vi "Is Enum Control.vi"(8 "error in":errorcluster, 11 "control reference in":refnum<vi>) -> (0 "error out":errorcluster, 1 "is enum control":bool, 2 "enum reference out":refnum<vi>, 3 "control reference out":refnum<vi>)   [LabVIEW 2020, in "Plug-In SDK Measurement.lvlib"]
uses:
  Plug-In SDK Measurement.lvlib
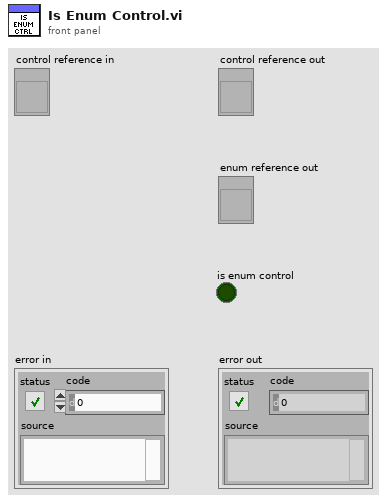
[diagram p1: front panel]
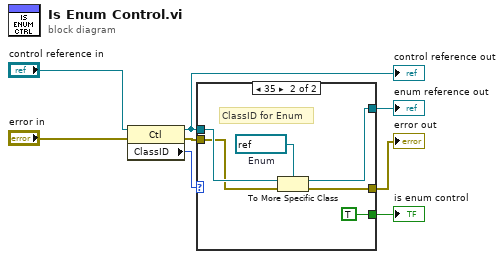
[diagram p0: block diagram]
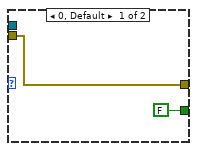
[diagram p2: hidden frame]
diagram:
  n1 = property class="Ctl"(reference="control reference in", error in="error in") -> (reference out=w4:refnum<vi>, error out=w3:errorcluster, "ClassID"=w8:u32)
  "control reference out" <- w4
  n2 = case shown="35" w8 {
    tunnel: [FALSE TRUE] -> w5
    tunnel: w4 -> [_ w14]
    tunnel: w3 -> [w9 w13]
    tunnel: [w9 w12] -> w2
    tunnel: [_ w11] -> w1
    frame 0, Default {
    }
    frame 35 {
      w15 = refnum<vi> refnum  # Enum
      # "ClassID for Enum"
      n3 = To More Specific Class(target class=w15, reference=w14, error in=w13) -> (specific class reference=w11:refnum<vi>, error out=w12:errorcluster)
    }
  }
  "is enum control" <- w5
  "error out" <- w2
  "enum reference out" <- w1
